vi "SSL Detection Ball.vi"(5 "Time Stamp":timestamp, 8 "error in":errorcluster, 9 "Array":u8[](array[numeric]) format="%02x") -> (0 "error out":errorcluster, 1 "Length-delimited":u8[](array[numeric]) format="%02x", 3 "Detection Ball":refnum<class "Ball.lvclass">)   [LabVIEW 2018]
uses:
  Ball_class/Ball.lvclass
  C:/Users/anton/Desktop/roboime/oop-vision/SSL_AI/Object_class/Object.lvclass
  Object_class/Object.lvclass/Object.ctl
  Ball_class/Ball.lvclass/Ball.ctl
  Object_class/Write x.vi
  Object_class/Write y.vi
  Ball_class/Write Valid.vi
  Varint Decoder uint32.vi
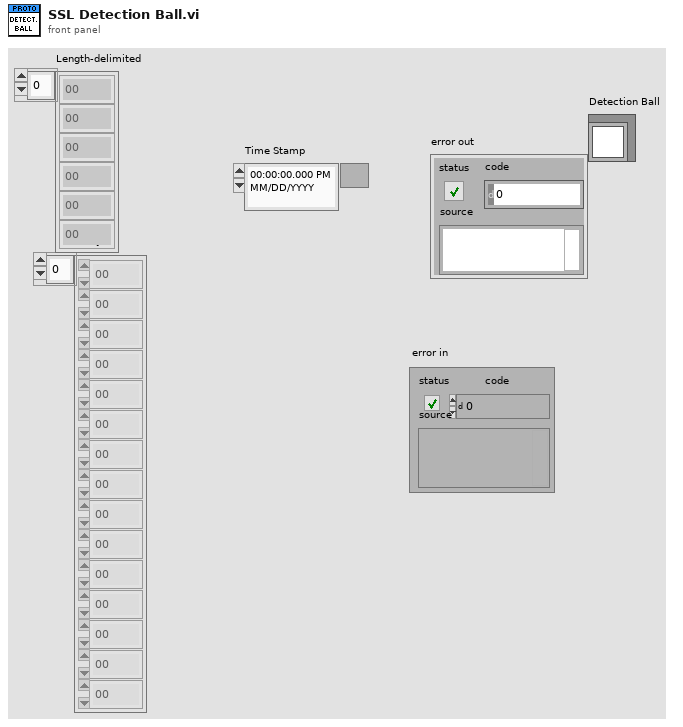
[diagram p1: front panel]
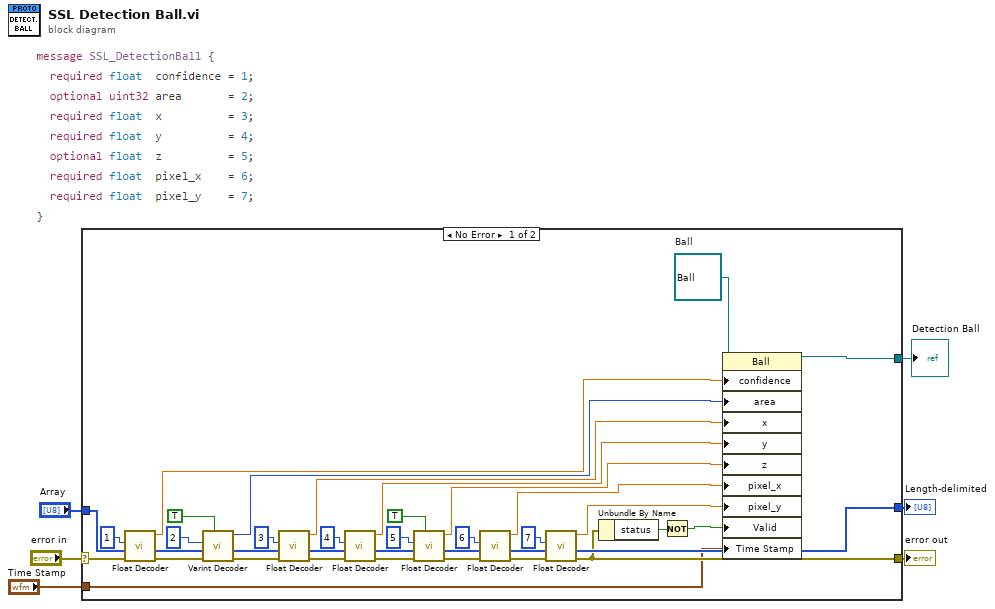
[diagram p0: block diagram]
diagram:
  n1 = case shown="No Error" "error in" {
    selector: "error in" -> [w42 w45]
    tunnel: [w19 w45] -> w5
    tunnel: [w29 w44] -> w4
    tunnel: "Array" -> [w21 w44]
    tunnel: "Time Stamp" -> [w8 _]
    tunnel: [w7 _] -> w1
    frame No Error {
      w17 = refnum<class "Ball.lvclass"> refnum  # Ball
      n2 = call "Float Decoder.vi"("error in (no error)"=w42, "Array"=w21, "Key"=1) -> ("error out"=w41:errorcluster, "array w/ subset deleted"=w22:u8[], "Float"=w16:sgl)  [unwired: 5 in, 1 out]
      n3 = call-poly "Varint Decoder.vi"("Optional"=TRUE, "error in (no error)"=w41, "Array"=w22, "Key"=2) -> ("error out"=w40:errorcluster, "array w/ subset deleted"=w23:u8[], "Varint"=w15:u32)  [unwired: 4 in, 1 out]
      n4 = call "Float Decoder.vi"("error in (no error)"=w40, "Array"=w23, "Key"=3) -> ("error out"=w39:errorcluster, "array w/ subset deleted"=w24:u8[], "Float"=w14:sgl)  [unwired: 5 in, 1 out]
      n5 = call "Float Decoder.vi"("error in (no error)"=w39, "Array"=w24, "Key"=4) -> ("error out"=w34:errorcluster, "array w/ subset deleted"=w25:u8[], "Float"=w13:sgl)  [unwired: 5 in, 1 out]
      n6 = call "Float Decoder.vi"("Optional"=TRUE, "error in (no error)"=w34, "Array"=w25, "Key"=5) -> ("error out"=w32:errorcluster, "array w/ subset deleted"=w27:u8[], "Float"=w12:sgl)  [unwired: 4 in, 1 out]
      n7 = call "Float Decoder.vi"("error in (no error)"=w32, "Array"=w27, "Key"=6) -> ("error out"=w30:errorcluster, "array w/ subset deleted"=w28:u8[], "Float"=w11:sgl)  [unwired: 5 in, 1 out]
      n8 = call "Float Decoder.vi"("error in (no error)"=w30, "Array"=w28, "Key"=7) -> ("error out"=w19:errorcluster, "array w/ subset deleted"=w29:u8[], "Float"=w10:sgl)  [unwired: 5 in, 1 out]
      n9 = Unbundle By Name(w19) -> ("status"=w18:bool)
      n10 = Not(x=w18) -> (.not. x?=w9:bool)
      n11 = property class="Ball"(reference=w17, "confidence"=w16, "area"=w15, "x"=w14, "y"=w13, "z"=w12, "pixel_x"=w11, "pixel_y"=w10, "Valid"=w9, "Time Stamp"=w8) -> (reference out=w7:refnum<class "Ball.lvclass">)  [unwired: 1 in, 1 out]
    }
    frame Error {
    }
  }
  "error out" <- w5
  "Length-delimited" <- w4
  "Detection Ball" <- w1
